vi "OTDR.vi"(0 "Res BW Units":enum16{"PM", "GHz"}(ring)=enum."GHz") -> (5 "Settings Applied?":bool)   [LabVIEW 2012]
uses:
  bin/OVA32.dll
panel:
  in  "StartCheck":bool=TRUE
  out "accepted?":bool
  in  "Sync Matrix Windows":bool
  in  "X2":dbl format="%.4f"
  in  "X1":dbl format="%.4f"
  out "arraySize":u32
  out "Grp Index Buf":dbl=1.5 format="%.2f"
  out "X-Units Buf":u16
  out "divisor":dbl format="%.6f"
  out "length inc(m)":dbl format="%.2f"
  in  "Group Index":dbl=1.5 format="%.2f"
  out "X Buffer":u16(ring) items=["Time (ns)", "Length (m)"]
  in  "X-Units":u16(ring) items=["Time (ns)", "Length (m)"]
  out "Retain Buffer":bool
  out "window chgd?":bool
  out "Reinit?":bool
  out "curr matrix":string
  out "timeInc (ns)":dbl format="%.2f"
  out "t_max":dbl format="%.2f"
  out "Prev Matrix Sel":i32
  in  "States":T1(ring)
  in  "Retain Settings":bool
  in  "Matrix Sel":i32(ring) caption="Matrix to View/Window" items=["A", "B", "C"]
  out "Graph":cluster{"X0":dbl, "dX":dbl, "Data":dbl[][]}(graph) caption="Time Domain Impulse Response of Matrix A"
  in  "Cancel":bool
  out "cancelled?":bool
  in  "accept":bool
  out "Res. BW":dbl=838.8608 caption="Window Res BW (pm)" format="%.2f"
  in  "Sigma (ns)":dbl=0.0005 min=0.0005 max=1.0 format="%.3f"
  # "OVA Time Domain Windowing"
  # "Window Parameters"
  # "Cursor Positions"
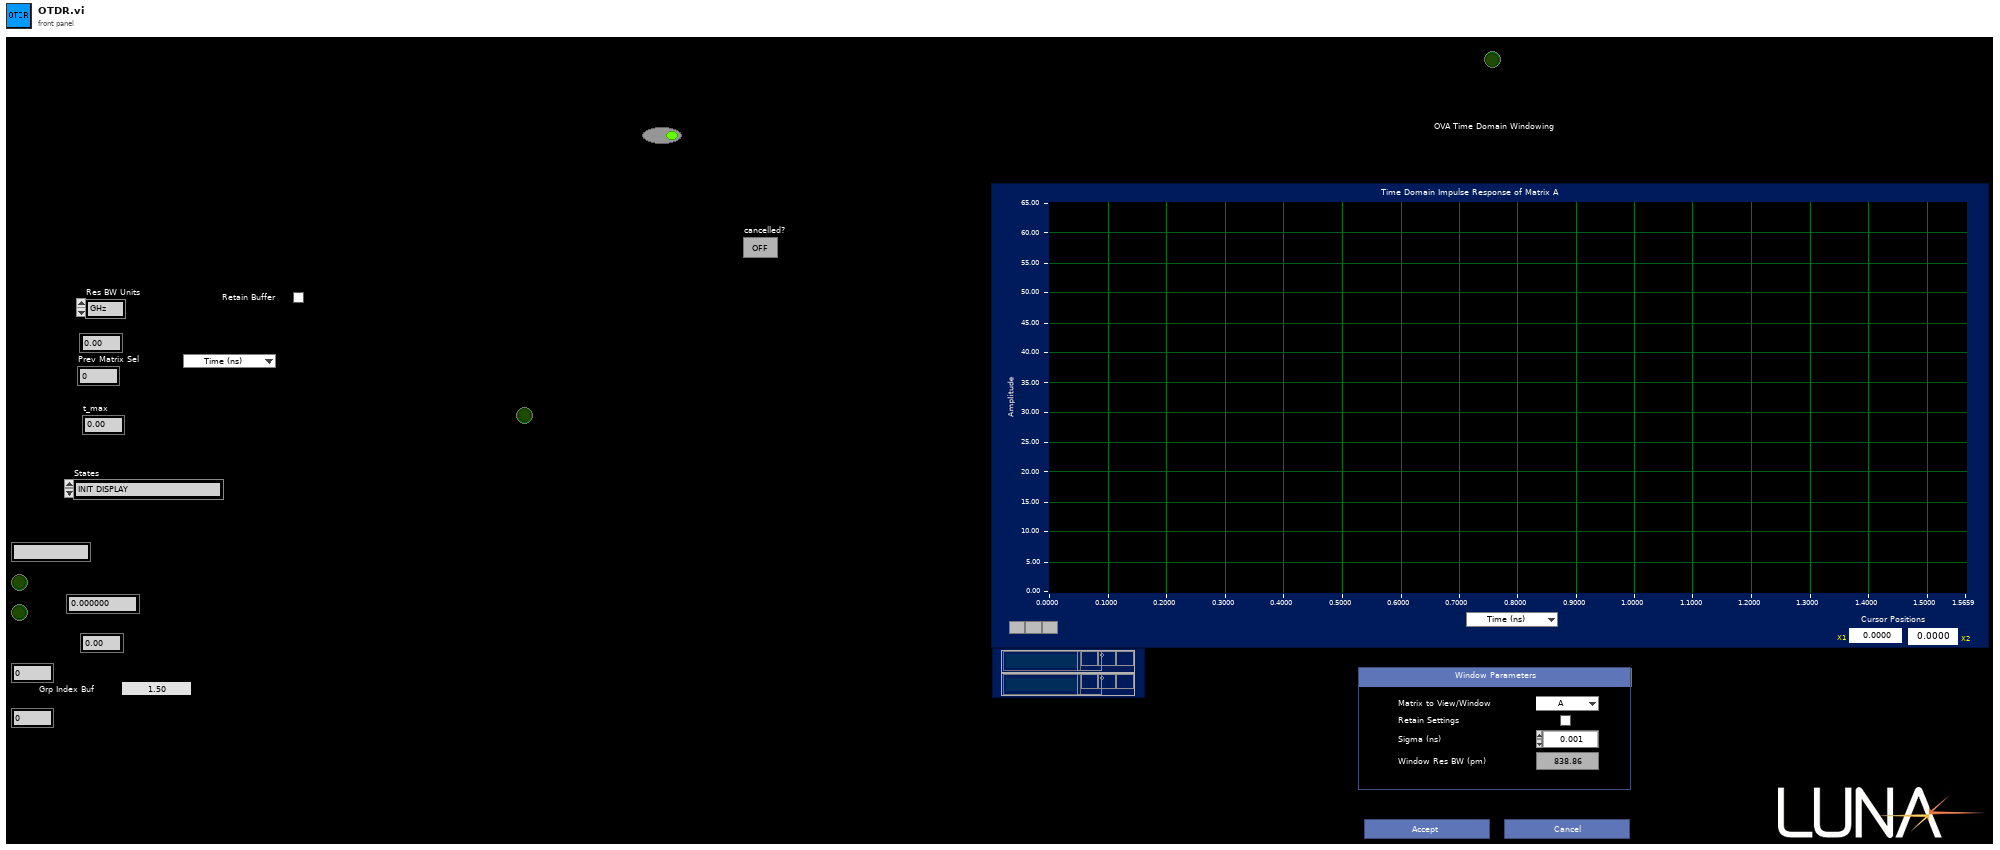
[diagram p1: front panel]
types:
  T1 = enum16{"INIT DISPLAY", "INIT SYSTEM", "CHANGE X AXIS", "WINDOW OTDR", "POST PROCESSING"}
  T2 = enum16{"NONE", "MB_ICONHAND", "MB_ICONQUESTION", "MB_ICONEXCLAMATION", "MB_ICONINFORMATION"}
  T3 = enum16{"MB_OK", "MB_OKCANCEL", "MB_ABORTRETRYIGNORE", "MB_YESNOCANCEL", "MB_YESNO", "MB_RETRYCANCEL"}
  T4 = cluster{"dutLength":dbl, "endWL":dbl, "segSize":u32, "measType":u8, "avgDisp":dbl, "sampleSpacing":dbl, "startFreq":dbl, "timeInc":dbl, "tdWinResBWGHz":dbl, "numAvgs":u32, "timeStr":string, "Pulse Cmp Enabled?":bool, "dispReferenceWL":dbl, "dsprsnSlope":dbl, "device Name":string, "file Name":string}
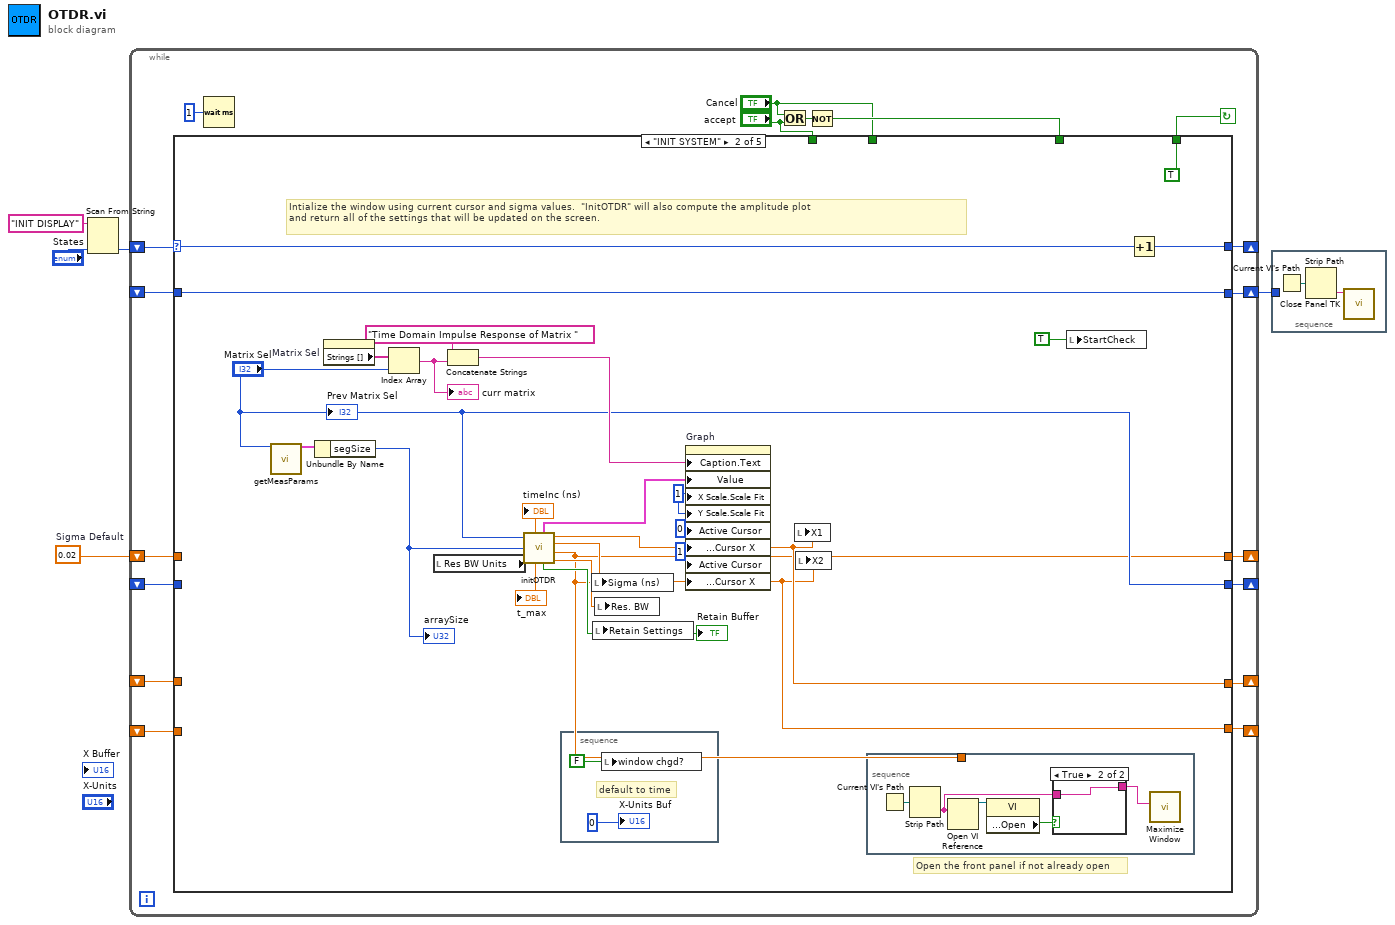
[diagram p0: block diagram]
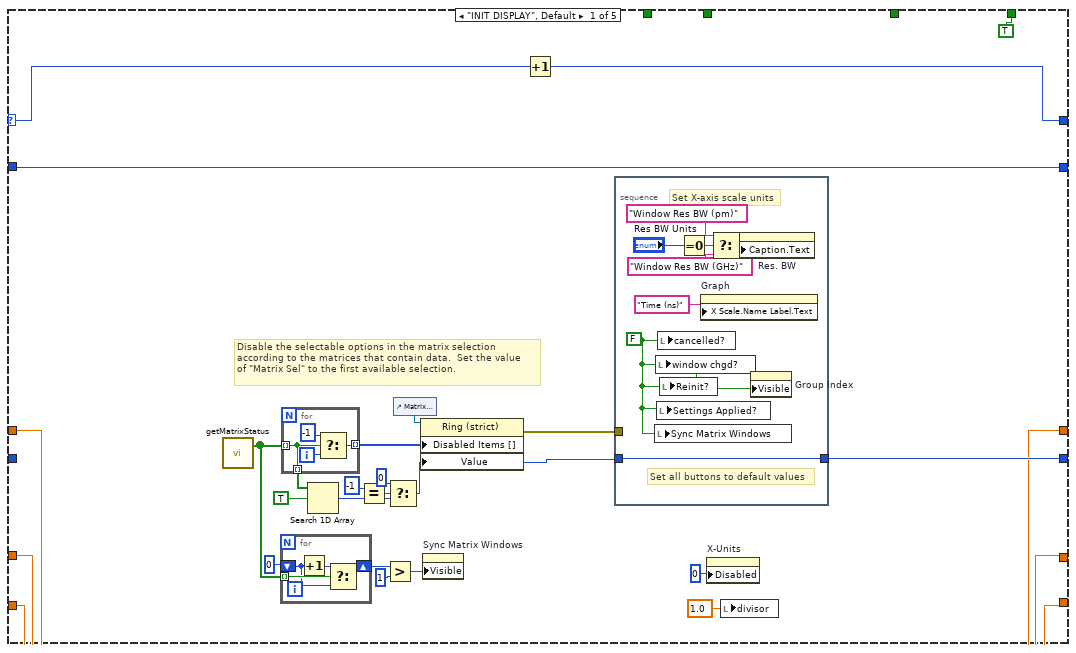
[diagram p2: hidden frame]
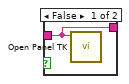
[diagram p3: hidden frame]
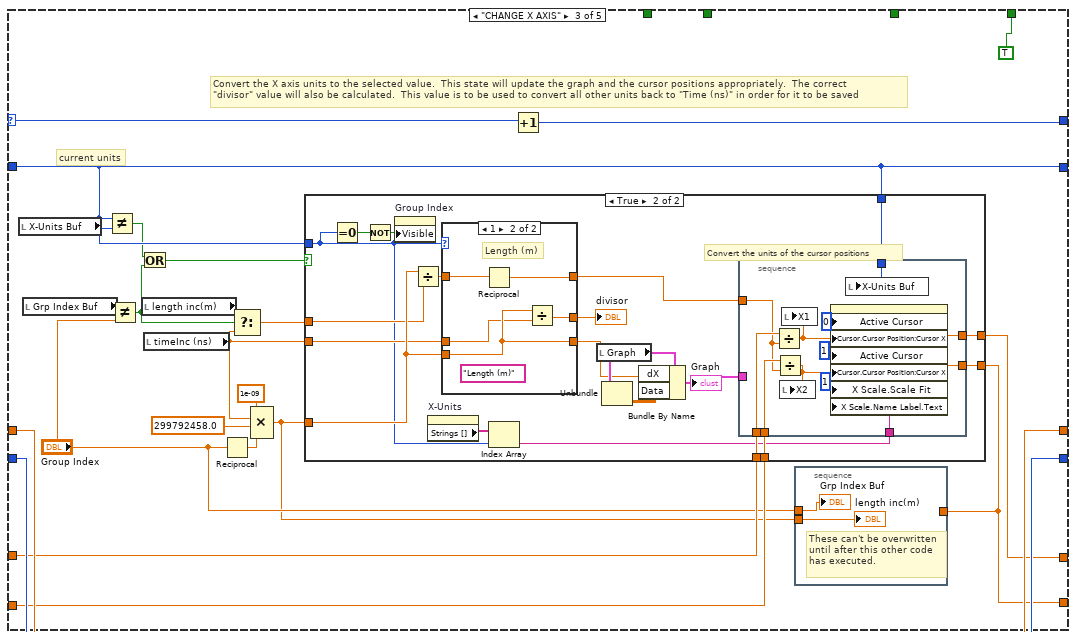
[diagram p4: hidden frame]
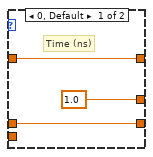
[diagram p6: hidden frame]
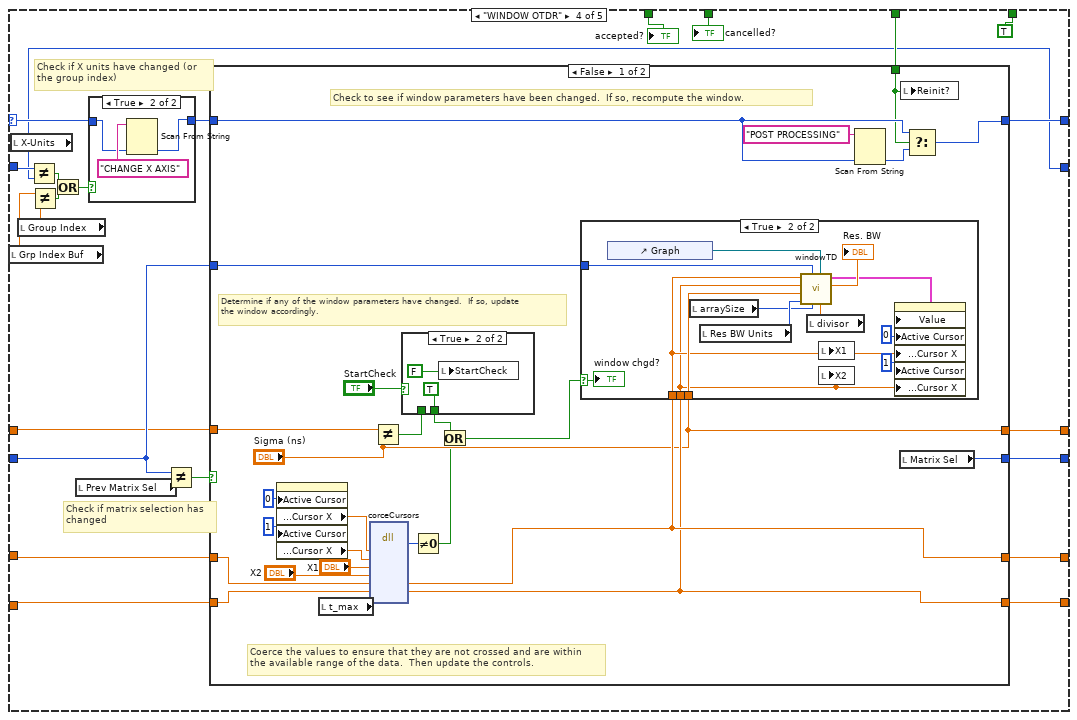
[diagram p7: hidden frame]
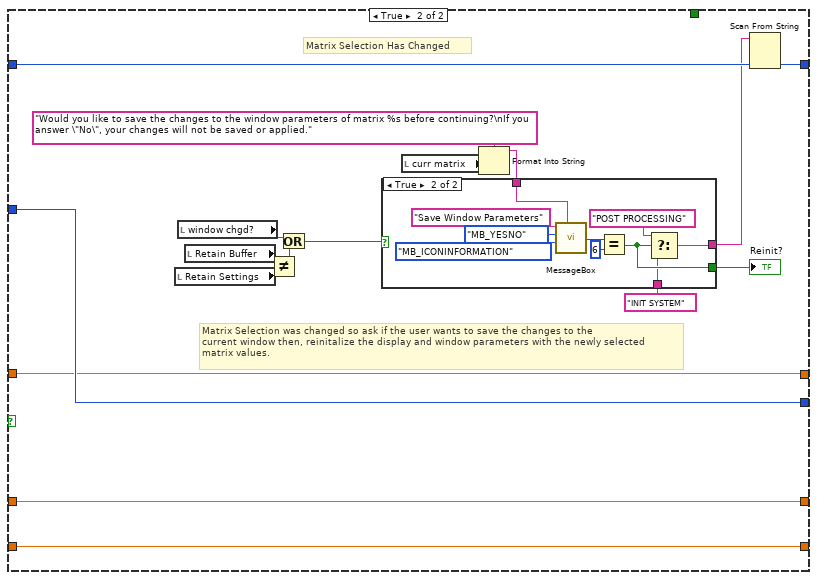
[diagram p11: hidden frame]
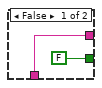
[diagram p12: hidden frame]
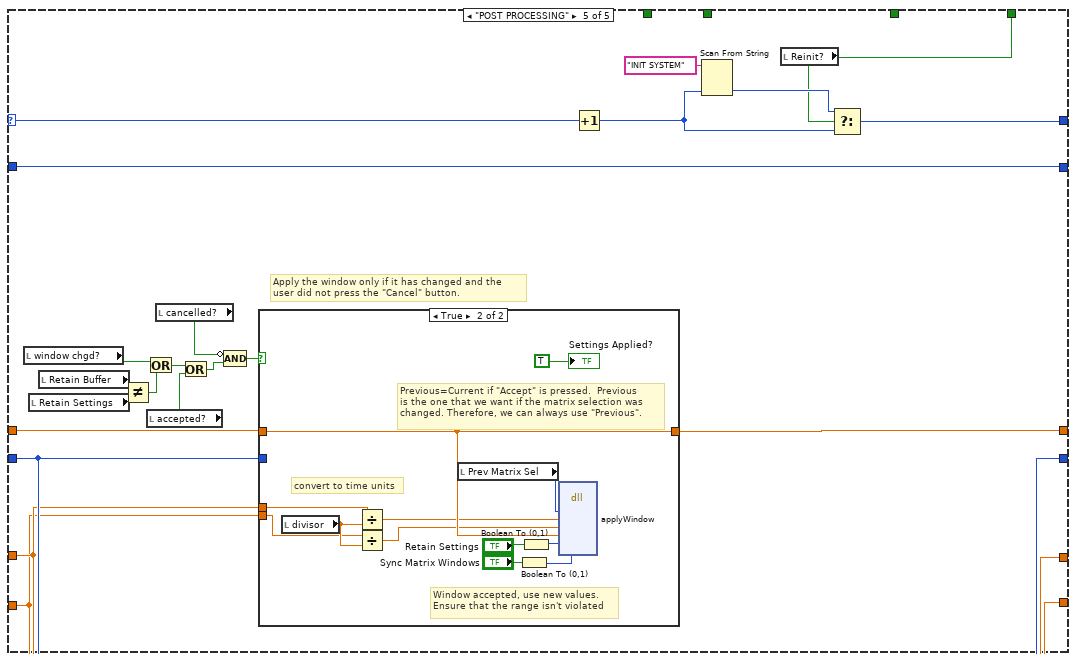
[diagram p13: hidden frame]
diagram:
  w2 = 0.02  # Sigma Default
  n1 = Scan From String(input string="INIT DISPLAY" ("Input String"), default 1="States") -> (output 1=w3:T1)  [unwired: 3 in, 3 out]
  n2 = while {
    shift-right: [w14] -> _
    shift-left: w3 -> [w23]
    shift-right: [w22] -> _
    shift-left: _ -> [w21]
    shift-right: [w20] -> _
    shift-left: w2 -> [w19]
    shift-right: [w17] -> _
    shift-left: _ -> [w16]
    shift-right: [w18] -> _
    shift-left: _ -> [w15]
    shift-right: [w7] -> w1
    shift-left: _ -> [w8]
    stop <- w12 continue-if-true
    n3 = Wait (ms)(milliseconds to wait=u32 1) -> ()  [unwired: 1 out]
    n4 = Or(x="Cancel", y="accept") -> (x .or. y?=w11:bool)
    n5 = Not(x=w11) -> (.not. x?=w10:bool)
    n6 = case shown="\"INIT SYSTEM\"" w23 {
      selector: w23 -> [w37 w75 w120 w172 w282]
      tunnel: [w36 w74 w119 w186 w276] -> w14
      tunnel: [w38 "Matrix Sel" w117 w185 w275] -> w22
      tunnel: w21 -> [_ _ w117 w184 w275]
      tunnel: [w33 w66 w116 w179 w278] -> w20
      tunnel: w19 -> [w33 _ w116 w178 w281]
      tunnel: [w35 w67 w106 w176 w267] -> w18
      tunnel: [w34 w68 w115 w177 w268] -> w17
      tunnel: w16 -> [w34 _ w114 w181 w268]
      tunnel: w15 -> [w35 _ w113 w180 w267]
      tunnel: [TRUE ("Reinit?") TRUE ("Reinit?") TRUE ("Reinit?") TRUE ("Reinit?") w266] -> w12
      tunnel: w10 -> [_ _ _ w174 _]
      tunnel: "Cancel" -> [_ _ _ w173 _]
      tunnel: w8 -> [w29 w73 w111 w170 w265]
      tunnel: [w29 w73 w111 w169 w265] -> w7
      tunnel: "accept" -> [_ _ _ w163 _]
      frame "INIT DISPLAY", Default {
        # "Disable the selectable options in the matrix selection\naccording to the matrices that contain data.  Set the value\nof \"Matrix Sel\" to the first available selection."
        n7 = call "getMatrixStatus.vi"() -> ("Meas Matrices Filled?"=w25:bool[])  [unwired: 5 in]
        n8 = for {
          tunnel: w25 -> [w52] mode=indexing
          shift-right: [w49] -> w27
          shift-left: 0 -> [w50]
          n9 = Increment(x=w50) -> (x+1=w51:i32)
          n10 = Select(t=w51, s=w52, f=w50) -> (s? t:f=w49:i32)
        }
        n11 = for {
          tunnel: [w56] -> w48 mode=indexing
          tunnel: [w55] -> w45 mode=indexing
          tunnel: w25 -> [w55] mode=indexing
          i -> [w54]
          n12 = Select(t=-1, s=w55, f=w54) -> (s? t:f=w56:i32)
        }
        n13 = Search 1D Array(1D array=w45, element=TRUE) -> (index of element=w42:i32)  [unwired: 1 in]
        n14 = Equal?(x=-1, y=w42) -> (x = y?=w44:bool)
        n15 = Greater?(x=w27, y=1) -> (0:w24:bool)
        n16 = Select(t=0, s=w44, f=w42) -> (s? t:f=w40:i32)
        n17 = control-ref of="Matrix Sel"() -> (w47:refnum<vi>)
        n18 = property class="Ring (strict)"(reference=w47, "Disabled Items []"=w48, "Value"=w40) -> (error out=w39:errorcluster)  [unwired: 1 in, 1 out]
        n19 = property on="Sync Matrix Windows" class="Bool (strict)"("Visible"=w24) -> ()  [unwired: 2 in, 2 out]
        n20 = Increment(x=w37) -> (x+1=w36:T1)
        n21 = stacked-sequence {
          tunnel: [w59] -> w38
          tunnel: w40 -> [w59]
          tunnel: w39 -> [_]
          frame #0 {
            w57 = FALSE
            # "Set all buttons to default values"
            # "Set X-axis scale units"
            n22 = local write "Sync Matrix Windows"(w57) -> ()
            n23 = local write "window chgd?"(w57) -> ()
            n24 = local write "Settings Applied?"(w57) -> ()
            n25 = local write "cancelled?"(w57) -> ()
            n26 = local write "Reinit?"(w57) -> ()
            n27 = Equal To 0?(x="Res BW Units") -> (x = 0?=w60:bool)
            n28 = property on="Graph" class="WFGraph (strict)"("X Scale.Name Label.Text"="Time (ns)") -> ()  [unwired: 2 in, 2 out]
            n29 = Select(t="Window Res BW (pm)", s=w60, f="Window Res BW (GHz)") -> (s? t:f=w63:string)
            n30 = property on="Res. BW" class="DigNum (strict)"("Caption.Text"=w63) -> ()  [unwired: 2 in, 2 out]
            n31 = property on="Group Index" class="DigNum (strict)"("Visible"=w57) -> ()  [unwired: 2 in, 2 out]
          }
        }
        n32 = property on="X-Units" class="Ring (strict)"("Disabled"=u8 0) -> ()  [unwired: 2 in, 2 out]
        n33 = local write "divisor"(1.0 ("multiplier")) -> ()
      }
      frame "INIT SYSTEM" {
        w84 = u8 1 ("Write Attribute")
        # "Open the front panel if not already open"
        # "Intialize the window using current cursor and sigma values.  \"InitOTDR\" will also compute the amplitude plot\nand return all of the settings that will be updated on the screen."
        n34 = call "getMeasParams.vi"("Matrix"="Matrix Sel") -> ("MeasParameters"=w70:T4)  [unwired: 13 in, 1 out]
        n35 = Unbundle By Name(w70) -> ("segSize"=w69:u32)
        "arraySize" <- w69
        n36 = property on="Matrix Sel" class="Ring (strict)"() -> ("Strings []"=w81:string[])  [unwired: 2 in, 2 out]
        n37 = Index Array(array=w81, index="Matrix Sel") -> (element=w80:string)
        "curr matrix" <- w80
        n38 = local read "Res BW Units"() -> (w87:enum16{"PM", "GHz"})
        n39 = Concatenate Strings("Time Domain Impulse Response of Matrix ", w80) -> (w82:string)
        n40 = call "initOTDR.vi"("matrix"="Matrix Sel", "matrixSize"=w69, "Res BW Units"=w87) -> ("timeInc (ns)"=→"timeInc (ns)":dbl, "t_max (ns)"=→"t_max":dbl, "Windowed JM Cluster"=w76:cluster{"X0":dbl, "dX":dbl, "Data":dbl[][]}, "Cursor X1"=w68:dbl, "Cursor X2"=w67:dbl, "Retain Settings"=w78:bool, "Sigma (ns)"=w66:dbl, "Res. BW"=w86:dbl)
        "Retain Buffer" <- w78
        n41 = stacked-sequence {
          frame #0 {
            # "default to time"
            n42 = local write "window chgd?"(FALSE ("window changed?")) -> ()
            "X-Units Buf" <- u16 0 ("X-Units Buf")
          }
        }
        n43 = local write "Sigma (ns)"(w66) -> ()
        n44 = local write "Retain Settings"(w78) -> ()
        n45 = local write "Res. BW"(w86) -> ()
        n46 = property on="Graph" class="WFGraph (strict)"("Caption.Text"=w82, "Value"=w76, "X Scale.Scale Fit"=w84, "Y Scale.Scale Fit"=w84, "Active Cursor"=u32 0, "Cursor.Cursor Position:Cursor X"=w68, "Active Cursor"=u32 1, "Cursor.Cursor Position:Cursor X"=w67) -> ()  [unwired: 2 in, 2 out]
        n47 = local write "X1"(w68) -> ()
        n48 = local write "X2"(w67) -> ()
        n49 = stacked-sequence {
          tunnel: w66 -> [_]
          frame #0 {
            n50 = Current VI's Path() -> (path=w94:path)
            n51 = Strip Path(path=w94) -> (name=w92:string)  [unwired: 1 out]
            n52 = Open VI Reference(vi path=w92) -> (vi reference=w95:refnum<vi>)  [unwired: 5 in, 1 out]
            n53 = property class="VI"(reference=w95) -> ("Front Panel Window:Open"=w93:bool)  [unwired: 1 in, 2 out]
            n54 = case shown="True" w93 {
              tunnel: w92 -> [w96 w97]
              tunnel: [w96 w97] -> w91
              frame False {
                n55 = call "Open Panel TK.vi"("VI name"=w96) -> ()  [unwired: 10 in, 1 out]
              }
              frame True {
              }
            }
            n56 = call "Maximize Window.vi"("window name  (\"\")"=w91) -> ()  [unwired: 5 in, 2 out]
          }
        }
        n57 = local write "StartCheck"(TRUE ("StartCheck")) -> ()
        n58 = Increment(x=w75) -> (x+1=w74:T1)
        "Prev Matrix Sel" <- "Matrix Sel"
      }
      frame "CHANGE X AXIS" {
        # "Convert the X axis units to the selected value.  This state will update the graph and the cursor positions appropriately.  The correct\n\"divisor\" value will also be calculated.  This value is to be used to convert all other units back to \"Time (ns)\" in order for it to be saved"
        # "current units"
        n59 = local read "X-Units Buf"() -> (w112:u16)
        n60 = local read "Grp Index Buf"() -> (w103:dbl)
        n61 = Not Equal?(x=w111, y=w112) -> (x != y?=w104:bool)
        n62 = Not Equal?(x=w103, y="Group Index") -> (x != y?=w102:bool)
        n63 = Or(x=w104, y=w102) -> (x .or. y?=w105:bool)
        n64 = local read "length inc(m)"() -> (w98:dbl)
        n65 = local read "timeInc (ns)"() -> (w101:dbl)
        n66 = Reciprocal(x="Group Index") -> (1/x=w108:dbl)
        n67 = Select(t=w98, s=w102, f=w101) -> (s? t:f=w100:dbl)
        n68 = Compound Arithmetic op=MULTIPLY(1e-09, w101, 299792458.0 ("Input"), w108) -> (w99:dbl)
        n69 = case shown="True" w105 {
          tunnel: [w123 w139] -> w106
          tunnel: [w124 w138] -> w115
          tunnel: w114 -> [w124 w137]
          tunnel: w113 -> [w123 w136]
          tunnel: w111 -> [_ w126]
          tunnel: w111 -> [_ w135]
          tunnel: w99 -> [_ w130]
          tunnel: w101 -> [_ w129]
          tunnel: w100 -> [_ w128]
          frame False {
          }
          frame True {
            # "Convert the units of the cursor positions"
            n70 = Equal To 0?(x=w126) -> (x = 0?=w140:bool)
            n71 = Not(x=w140) -> (.not. x?=w142:bool)
            n72 = property on="Group Index" class="DigNum (strict)"("Visible"=w142) -> ()  [unwired: 2 in, 2 out]
            n73 = Divide(x=w130, y=w128) -> (x/y=w134:dbl)
            n74 = property on="X-Units" class="Ring (strict)"() -> ("Strings []"=w127:string[])  [unwired: 2 in, 2 out]
            n75 = case shown="1" w126 {
              tunnel: [w147 w151] -> w133
              tunnel: w134 -> [w147 w152]
              tunnel: [1.0 ("t") w150] -> w132
              tunnel: [w145 w149] -> w131
              tunnel: w129 -> [w145 w148]
              tunnel: w130 -> [_ w149]
              frame 0, Default {
                # "Time (ns)"
              }
              frame 1 {
                (unwired) "Length (m)"
                # "Length (m)"
                n76 = Reciprocal(x=w152) -> (1/x=w151:dbl)
                n77 = Divide(x=w149, y=w148) -> (x/y=w150:dbl)
              }
            }
            "divisor" <- w132
            n78 = Index Array(array=w127, index=w126) -> (element=w125:string)
            n79 = local read "Graph"() -> (w144:cluster{"X0":dbl, "dX":dbl, "Data":dbl[][]})
            n80 = Unbundle(w144) -> ("Data"=w141:dbl[][])  [unwired: 2 out]
            n81 = Bundle By Name(cluster=w144, "dX"=w131, "Data"=w141) -> (w143:cluster{"X0":dbl, "dX":dbl, "Data":dbl[][]})
            "Graph" <- w143
            n82 = stacked-sequence {
              tunnel: w143 -> [_]
              tunnel: [w155] -> w138
              tunnel: [w154] -> w139
              tunnel: w137 -> [w159]
              tunnel: w136 -> [w158]
              tunnel: w135 -> [w157]
              tunnel: w133 -> [w156]
              tunnel: w125 -> [w153]
              frame #0 {
                n83 = Divide(x=w159, y=w156) -> (x/y=w155:dbl)
                n84 = Divide(x=w158, y=w156) -> (x/y=w154:dbl)
                n85 = local write "X2"(w154) -> ()
                n86 = local write "X1"(w155) -> ()
                n87 = property on="Graph" class="WFGraph (strict)"("Active Cursor"=u32 0, "Cursor.Cursor Position:Cursor X"=w155, "Active Cursor"=u32 1, "Cursor.Cursor Position:Cursor X"=w154, "X Scale.Scale Fit"=u8 1, "X Scale.Name Label.Text"=w153) -> ()  [unwired: 2 in, 2 out]
                n88 = local write "X-Units Buf"(w157) -> ()
              }
            }
          }
        }
        n89 = Increment(x=w120) -> (x+1=w119:T1)
        n90 = stacked-sequence {
          tunnel: "Group Index" -> [w122]
          tunnel: w106 -> [_]
          tunnel: w99 -> [w121]
          frame #0 {
            # "These can't be overwritten\nuntil after this other code\nhas executed."
            "Grp Index Buf" <- w122
            "length inc(m)" <- w121
          }
        }
      }
      frame "WINDOW OTDR" {
        # "Check if matrix selection has\nchanged"
        # "Check if X units have changed (or\nthe group index)"
        # "X2"
        # "X1"
        n91 = local read "Grp Index Buf"() -> (w164:dbl)
        n92 = local read "X-Units"() -> (w169:u16)
        n93 = local read "Group Index"() -> (w168:dbl)
        n94 = Not Equal?(x=w170, y=w169) -> (x != y?=w166:bool)
        n95 = Not Equal?(x=w164, y=w168) -> (x != y?=w167:bool)
        n96 = Or(x=w166, y=w167) -> (x .or. y?=w165:bool)
        n97 = local read "Prev Matrix Sel"() -> (w183:i32)
        n98 = case shown="True" w165 {
          tunnel: w172 -> [w187 w189]
          tunnel: [w187 w188] -> w171
          frame False {
          }
          frame True {
            n99 = Scan From String(input string="CHANGE X AXIS" ("Input String"), default 1=w189) -> (output 1=w188:T1)  [unwired: 3 in, 3 out]
          }
        }
        n100 = Not Equal?(x=w184, y=w183) -> (x != y?=w182:bool)
        n101 = case shown="False" w182 {
          tunnel: w181 -> [w209 w247]
          tunnel: w180 -> [w208 w246]
          tunnel: [w206 w246] -> w176
          tunnel: w178 -> [w216 w238]
          tunnel: [w207 w247] -> w177
          tunnel: w184 -> [w215 w245]
          tunnel: w171 -> [w211 w249]
          tunnel: [w210 w248] -> w186
          tunnel: [w214 w245] -> w185
          tunnel: ["Sigma (ns)" w238] -> w179
          tunnel: w174 -> [w204 _]
          frame False {
            # "Determine if any of the window parameters have changed.  If so, update\nthe window accordingly."
            # "Coerce the values to ensure that they are not crossed and are within\nthe available range of the data.  Then update the controls."
            # "Check to see if window parameters have been changed.  If so, recompute the window."
            n102 = property on="Graph" class="WFGraph (strict)"("Active Cursor"=u32 0, "Active Cursor"=u32 1) -> ("Cursor.Cursor Position:Cursor X"=w199:dbl, "Cursor.Cursor Position:Cursor X"=w198:dbl)  [unwired: 2 in, 2 out]
            n103 = local read "t_max"() -> (w197:dbl)
            n104 = dll-call lib="C:/_src/OVA5000_DSP_falcon/Software/LabVIEW/OVA/SDK/OVA_5000_SDK_v5.14.3/bin/OVA32.dll" fn="corceCursors"("cursor1"=w199, "cursor2"=w198, "X1"="X1", "X2"="X2", "prevX1"=w209, "prevX2"=w208, "tMax"=w197) -> (w196:u8, "prevX1"=w207:dbl, "prevX2"=w206:dbl)  [unwired: 8 in, 2 out]
            n105 = Not Equal?(x=w216, y="Sigma (ns)") -> (x != y?=w192:bool)
            n106 = case shown="True" "StartCheck" {
              tunnel: [w217 TRUE] -> w193
              tunnel: w192 -> [w217 _]
              frame False {
              }
              frame True {
                n107 = local write "StartCheck"(FALSE) -> ()
              }
            }
            n108 = Not Equal To 0?(x=w196) -> (x != 0?=w194:bool)
            n109 = Or(x=w193, y=w194) -> (x .or. y?=w195:bool)
            n110 = case shown="True" w195 {
              selector: w195 -> [_ w228]
              tunnel: w215 -> [_ w230]
              tunnel: "Sigma (ns)" -> [_ w229]
              tunnel: w207 -> [_ w221]
              tunnel: w206 -> [_ w220]
              frame False {
              }
              frame True {
                n111 = control-ref of="Graph"() -> (w223:refnum<vi>)
                n112 = local read "arraySize"() -> (w222:u32)
                n113 = local read "Res BW Units"() -> (w232:enum16{"PM", "GHz"})
                n114 = local read "divisor"() -> (w224:dbl)
                n115 = call "windowTD.vi"("Divisor (conversion factor between units)"=w224, "Graph Ref"=w223, "MatrixSize"=w222, "Matrix Selected"=w230, "Units"=w232, "Sigma (ns)"=w229, "x2 (ns or m)"=w220, "x1 (ns or m)"=w221) -> ("Res. BW"=→"Res. BW":dbl, "Windowed JM Cluster"=w225:cluster{dbl, "time inc (ns)_":dbl, dbl[][]})  [unwired: 2 in]
                n116 = local write "X1"(w221) -> ()
                n117 = local write "X2"(w220) -> ()
                n118 = property on="Graph" class="WFGraph (strict)"("Value"=w225, "Active Cursor"=u32 0, "Cursor.Cursor Position:Cursor X"=w221, "Active Cursor"=u32 1, "Cursor.Cursor Position:Cursor X"=w220) -> ()  [unwired: 2 in, 2 out]
                "window chgd?" <- w228
              }
            }
            n119 = Scan From String(input string="POST PROCESSING" ("Input String"), default 1=w211) -> (output 1=w212:T1)  [unwired: 3 in, 3 out]
            n120 = local read "Matrix Sel"() -> (w214:i32)
            n121 = local write "Reinit?"(w204) -> ()
            n122 = Select(t=w211, s=w204, f=w212) -> (s? t:f=w210:T1)
          }
          frame True {
            # "Matrix Selection Has Changed"
            # "Matrix Selection was changed so ask if the user wants to save the changes to the\ncurrent window then, reinitalize the display and window parameters with the newly selected\nmatrix values."
            n123 = local read "Retain Settings"() -> (w237:bool)
            n124 = local read "window chgd?"() -> (w234:bool)
            n125 = local read "Retain Buffer"() -> (w236:bool)
            n126 = Not Equal?(x=w236, y=w237) -> (x != y?=w235:bool)
            n127 = Or(x=w234, y=w235) -> (x .or. y?=w233:bool)
            n128 = local read "curr matrix"() -> (w243:string)
            n129 = Format Into String(format string="Would you like to save the changes to the window parameters of matrix %s before continuing?\nIf you answer \"No\", your changes will not be saved or applied." ("message"), w243) -> (resulting string=w242:string)  [unwired: 2 in, 1 out]
            n130 = case shown="True" w233 {
              tunnel: w242 -> [_ w256]
              tunnel: [FALSE w255] -> w239
              tunnel: [w251 w253] -> w241
              tunnel: "INIT SYSTEM" ("Input String") -> [w251 w252]
              frame False {
              }
              frame True {
                n131 = call "MessageBox.vi"("message"=w256, "Icon Type"=T2."MB_ICONINFORMATION", "Button Types"=T3."MB_YESNO", "caption"="Save Window Parameters") -> ("Output Value"=w260:i32)  [unwired: 5 in]
                n132 = Equal?(x=w260, y=6) -> (x = y?=w255:bool)
                n133 = Select(t="POST PROCESSING" ("Input String"), s=w255, f=w252) -> (s? t:f=w253:string)
              }
            }
            "Reinit?" <- w239
            n134 = Scan From String(input string=w241, default 1=w249) -> (output 1=w248:T1)  [unwired: 3 in, 3 out]
          }
        }
        "cancelled?" <- w173
        "accepted?" <- w163
      }
      frame "POST PROCESSING" {
        # "Apply the window only if it has changed and the\nuser did not press the \"Cancel\" button."
        n135 = local read "window chgd?"() -> (w274:bool)
        n136 = local read "Retain Settings"() -> (w273:bool)
        n137 = local read "Retain Buffer"() -> (w272:bool)
        n138 = Not Equal?(x=w272, y=w273) -> (x != y?=w271:bool)
        n139 = Or(x=w274, y=w271) -> (x .or. y?=w264:bool)
        n140 = local read "accepted?"() -> (w262:bool)
        n141 = local read "cancelled?"() -> (w269:bool)
        n142 = Or(x=w264, y=w262) -> (x .or. y?=w263:bool)
        n143 = Compound Arithmetic op=AND(invert w269, w263) -> (w270:bool)
        n144 = case shown="True" w270 {
          tunnel: [w283 w293] -> w278
          tunnel: w281 -> [w283 w293]
          tunnel: w275 -> [_ _]
          tunnel: w268 -> [_ w289]
          tunnel: w267 -> [_ w288]
          frame False {
            # "Cancelled"
          }
          frame True {
            # "convert to time units"
            # "Previous=Current if \"Accept\" is pressed.  Previous\nis the one that we want if the matrix selection was \nchanged. Therefore, we can always use \"Previous\"."
            # "Window accepted, use new values. \nEnsure that the range isn't violated"
            n145 = local read "divisor"() -> (w290:dbl)
            n146 = Divide(x=w289, y=w290) -> (x/y=w287:dbl)
            n147 = Divide(x=w288, y=w290) -> (x/y=w286:dbl)
            n148 = local read "Prev Matrix Sel"() -> (w292:i32)
            n149 = Boolean To (0,1)(Boolean="Sync Matrix Windows") -> (0, 1=w284:i16)
            n150 = Boolean To (0,1)(Boolean="Retain Settings") -> (0, 1=w294:i16)
            n151 = dll-call lib="C:/_src/OVA5000_DSP_falcon/Software/LabVIEW/OVA/SDK/OVA_5000_SDK_v5.14.3/bin/OVA32.dll" fn="applyWindow"("matrix"=w292, "cursor1"=w287, "curosor2"=w286, "sigma"=w293, "save"=w294, "sync"=w284) -> ()  [unwired: 10 in, 2 out]
            "Settings Applied?" <- TRUE ("Settings Applied?")
          }
        }
        n152 = Increment(x=w282) -> (x+1=w277:T1)
        n153 = Scan From String(input string="INIT SYSTEM" ("Input String"), default 1=w277) -> (output 1=w279:T1)  [unwired: 3 in, 3 out]
        n154 = local read "Reinit?"() -> (w266:bool)
        n155 = Select(t=w279, s=w266, f=w277) -> (s? t:f=w276:T1)
      }
    }
  }
  n156 = stacked-sequence {
    tunnel: w1 -> [_]
    frame #0 {
      n157 = Current VI's Path() -> (path=w297:path)
      n158 = Strip Path(path=w297) -> (name=w296:string)  [unwired: 1 out]
      n159 = call "Close Panel TK.vi"("VI name"=w296) -> ()  [unwired: 10 in, 1 out]
    }
  }
